vi "Read configuration.vi"(8 "error in":errorcluster, 11 "PLTarget cDAQ in":refnum<class "PLTarget PXI.lvclass">) -> (0 "error out":errorcluster, 2 "configuration":refnum<class "NISE_CEF_serializable configuration.lvclass">, 3 "PLTarget cDAQ out":refnum<class "PLTarget PXI.lvclass">)   [LabVIEW 2013, in "PLTarget PXI.lvclass"]
uses:
  PLTarget PXI.lvclass
  <vilib>/NI/Configuration Framework/serializable configuration/NISE_CEF_serializable configuration.lvclass
  PLTarget PXI.lvclass/PLTarget PXI.ctl
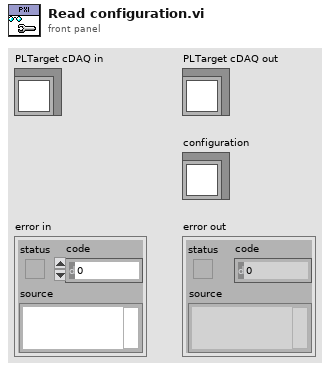
[diagram p1: front panel]
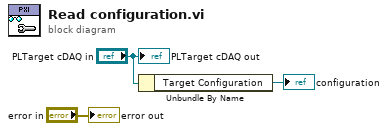
[diagram p0: block diagram]
diagram:
  n1 = Unbundle By Name("PLTarget cDAQ in") -> ("Target Configuration"=→"configuration":refnum<class "PL_Target Configuration.lvclass">)
  "error out" <- "error in"
  "PLTarget cDAQ out" <- "PLTarget cDAQ in"
